vi "CalculaNumeroCiclosBurst.vi"(1 "ms_burst":dbl, 2 "frec":dbl=4000.0 format="%#_13g") -> (0 "# ciclos":i32)   [LabVIEW 2019, in "Prueba08.lvclass"]
uses:
  Prueba08.lvclass
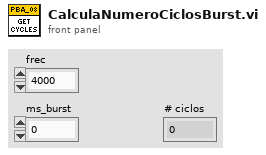
[diagram p1: front panel]
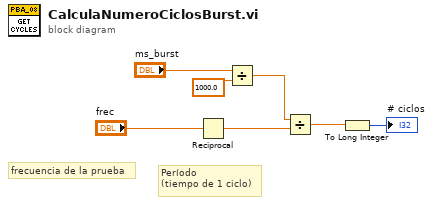
[diagram p0: block diagram]
diagram:
  # "frecuencia de la prueba"
  # "Período\n(tiempo de 1 ciclo)"
  n1 = Reciprocal(x="frec") -> (1/x=w4:dbl)
  n2 = Divide(x="ms_burst", y=1000.0) -> (x/y=w1:dbl)
  n3 = Divide(x=w1, y=w4) -> (x/y=w6:dbl)
  n4 = To Long Integer(number=w6) -> (32bit integer=→"# ciclos":i32)
